vi "CaseStructure to Code.vi"(8 "error in":errorcluster, 10 "Frames code[]":string[](array[string]), 11 "case struct ref.":refnum<vi>) -> (0 "error out":errorcluster, 2 "C code":string, 3 "terminals info":T1)   [LabVIEW 2014]
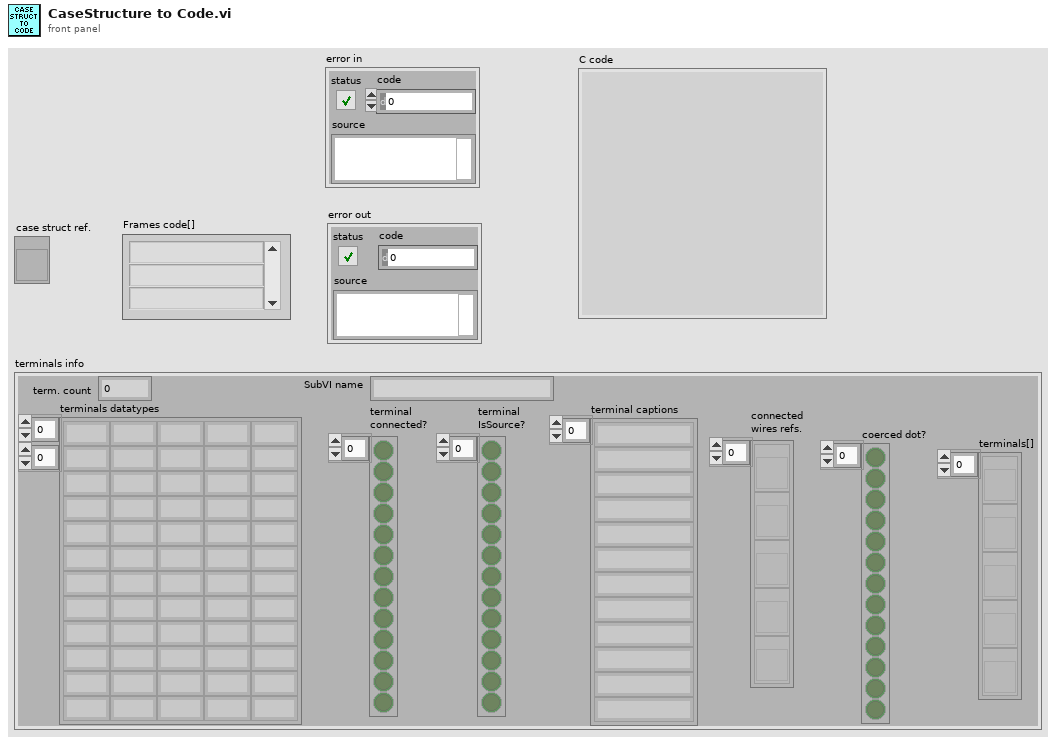
[diagram p1: front panel]
types:
  T1 = cluster{"terminals datatypes":string[][], "terminal\nconnected?":bool[], "terminal captions":string[], "term. count":i32, "terminal\nIsSource?":bool[], "SubVI name":string, "connected\nwires refs.":refnum<vi>[], "coerced dot?":bool[], "terminals[]":refnum<vi>[]}
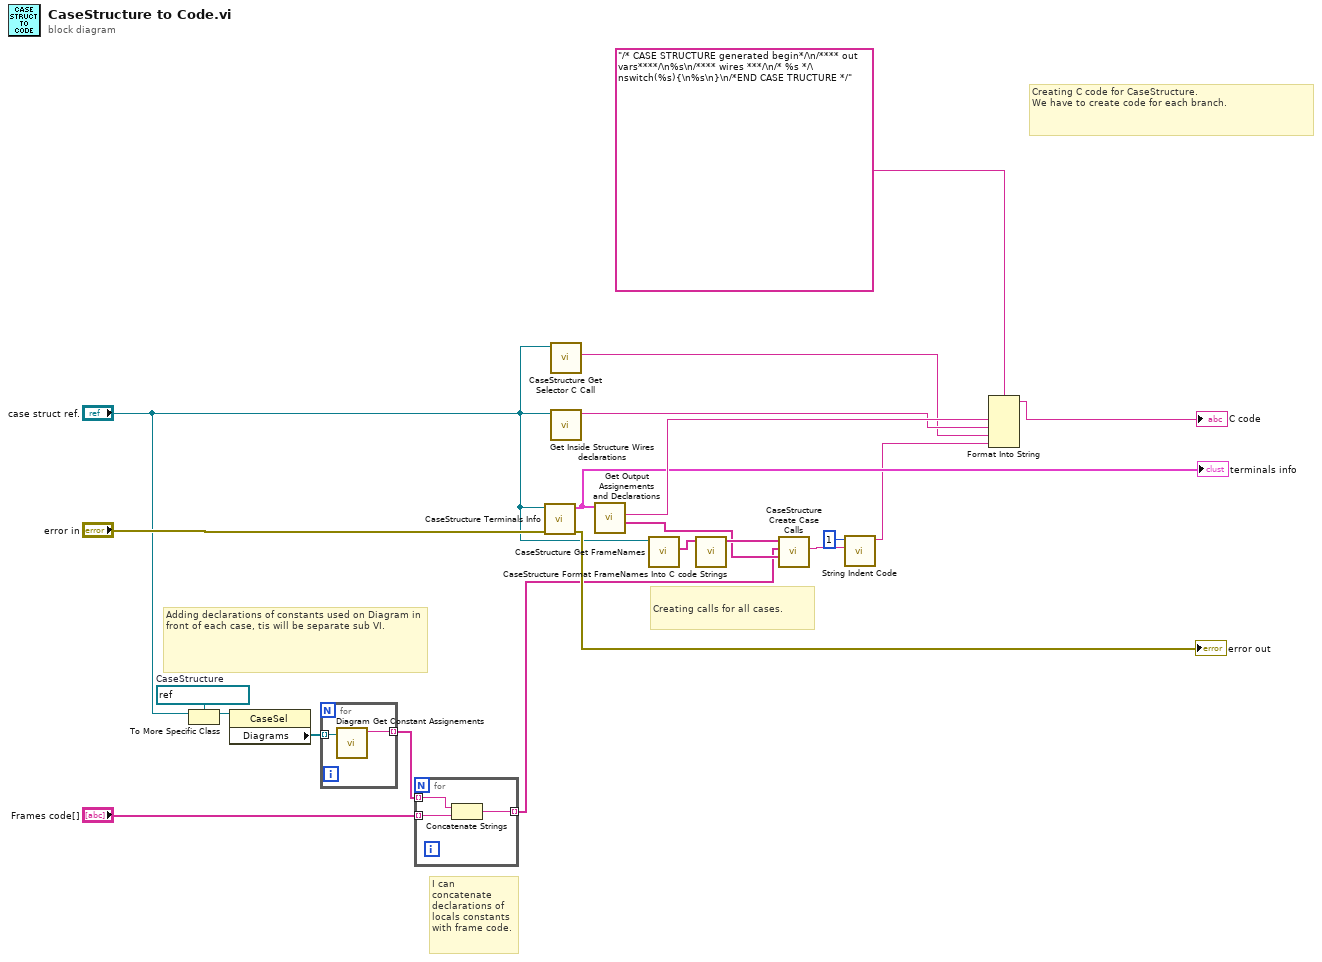
[diagram p0: block diagram]
diagram:
  w8 = refnum<vi> refnum  # CaseStructure
  # "I can concatenate declarations of locals constants with frame code."
  # "Adding declarations of constants used on Diagram in front of each case, tis will be separate sub VI."
  # "Creating calls for all cases."
  # "Creating C code for CaseStructure.\nWe have to create code for each branch."
  n1 = To More Specific Class(target class=w8, reference="case struct ref.") -> (specific class reference=w7:refnum<vi>)  [unwired: 1 in, 1 out]
  n2 = property class="CaseSel"(reference=w7) -> ("Diagrams"=w5:refnum<vi>[])  [unwired: 1 in, 2 out]
  n3 = for {
    tunnel: w5 -> [w23] mode=indexing
    tunnel: [w22] -> w2 mode=indexing
    n4 = call "Diagram Get Constant Assignements.vi"("Diagram ref."=w23) -> ("Constant assignements to wires"=w22:string)  [unwired: 10 in]
  }
  n5 = for {
    tunnel: w2 -> [w25] mode=indexing
    tunnel: "Frames code[]" -> [w26] mode=indexing
    tunnel: [w24] -> w3 mode=indexing
    n6 = Concatenate Strings(w25, w26) -> (w24:string)
  }
  n7 = call "CaseStructure Terminals Info.vi"("error in"="error in", "case structure ref."="case struct ref.") -> ("error out"=→"error out":errorcluster, "output cluster"=w17:T1)  [unwired: 8 in]
  "terminals info" <- w17
  n8 = call "CaseStructure Get Selector C Call.vi"("GObject in"="case struct ref.") -> ("CaseSelector connected wire name"=w13:string)  [unwired: 9 in, 1 out]
  n9 = call "Get Inside Structure Wires declarations.vi"("GObject in"="case struct ref.") -> ("structure inside wires C declarations"=w16:string)  [unwired: 10 in]
  n10 = call "Get Output Assignements and Declarations.vi"("output cluster"=w17) -> ("output assignements, for multiframes"=w12:string[], "output declarations"=w18:string)  [unwired: 8 in, 1 out]
  n11 = call "CaseStructure Get FrameNames.vi"("GObject in"="case struct ref.") -> ("Frame Names"=w15:string[])  [unwired: 8 in, 2 out]
  n12 = call "CaseStructure Format FrameNames Into C code Strings.vi"("FrameNames in"=w15) -> ("c code cases names"=w14:string[])  [unwired: 10 in]
  n13 = call "CaseStructure Create Case Calls.vi"("Output variables assignements"=w12, "Frames code[]"=w3, "FrameNames in"=w14) -> ("Switch Cases C calls all as string"=w11:string)  [unwired: 7 in, 1 out]
  n14 = call "String Indent Code.vi"("complete code"=w11, "actual nested level"=1) -> ("indented code"=w9:string)  [unwired: 9 in]
  n15 = Format Into String(format string="/* CASE STRUCTURE generated begin*/\n/**** out vars****/\n%s\n/**** wires ***/\n/* %s */\nswitch(%s){\n%s\n}\n/*END CASE TRUCTURE */", w18, w16, w13, w9) -> (resulting string=→"C code":string)  [unwired: 2 in, 1 out]
